vi "Dye Settings.vi"(6 "New Dye":bool, 8 "error in (no error)":errorcluster, 11 "Settings in":refnum<class "Settings.lvclass">=refnum) -> (0 "error out":errorcluster, 1 "Changed":bool, 2 "Pulse Sequence":T1(array[cluster])=[{"LED Name"="Cyan (488 nm)", "Pulse Length (s)"=0.1, "Delay Before (s)"=0.0, "Delay After (s)"=0.1, "Trigger Camera"=FALSE}, {"LED Name"="Red 2 (636 nm)", "Pulse Length (s)"=0.2, "Delay Before (s)"=0.0, "Delay After (s)"=0.1, "Trigger Camera"=TRUE}], 3 "Settings out":refnum<class "Settings.lvclass">)   [LabVIEW 2010, in "Settings.lvclass"]
uses:
  Settings.lvclass
  Settings.lvclass/Settings.ctl
panel:
  in  "# Pulses":i32=5 min=1 max=100
  out "Input OK":bool
  in  "Dye Name":string="Alexa 488"
  in  "Exposure (s)":dbl=0.2 min=0.0001 max=5.0
  in  "Delay After (s) 2":dbl=0.1 min=0.001 max=10.0 step=0.001
  in  "Pulse Length (s) 2":dbl=0.2 min=0.001 max=10.0 step=0.001
  in  "Delay Before (s) 2":dbl min=0.0 max=10.0 step=0.001
  in  "Delay After (s)":dbl=0.1 min=0.001 max=10.0 step=0.001
  in  "Pulse Length (s)":dbl=0.1 min=0.001 max=10.0 step=0.001
  in  "Delay Before (s)":dbl min=0.0 max=10.0 step=0.001
  out "XY Graph":cluster{dbl[], dbl[]}[](graph)=[{[0.0, 0.0, 0.0, 0.1, 0.1, 1.7000000000000002], [0.0, 0.0, 1.0, 1.0, 0.0, 0.0]}, {[0.0, 0.2, 0.2, 0.4, 0.4, 0.5, 0.5, 0.5, 0.7, 0.7, 0.7999999999999999, 0.7999999999999999, 0.7999999999999999, 1.0, 1.0, 1.1, 1.1, 1.1, 1.3, 1.3, 1.4000000000000001, 1.4000000000000001, 1.4000000000000001, 1.6, 1.6, 1.7000000000000002], [0.0, 0.0, 1.0, 1.0, 0.0, 0.0, 0.0, 1.0, 1.0, 0.0, 0.0, 0.0, 1.0, 1.0, 0.0, 0.0, 0.0, 1.0, 1.0, 0.0, 0.0, 0.0, 1.0, 1.0, 0.0, 0.0]}, {[0.0, 0.2, 0.2, 0.4, 0.4, 0.5, 0.5, 0.5, 0.7, 0.7, 0.7999999999999999, 0.7999999999999999, 0.7999999999999999, 1.0, 1.0, 1.1, 1.1, 1.1, 1.3, 1.3, 1.4000000000000001, 1.4000000000000001, 1.4000000000000001, 1.6, 1.6, 1.7000000000000002], [0.0, 0.0, 1.0, 1.0, 0.0, 0.0, 0.0, 1.0, 1.0, 0.0, 0.0, 0.0, 1.0, 1.0, 0.0, 0.0, 0.0, 1.0, 1.0, 0.0, 0.0, 0.0, 1.0, 1.0, 0.0, 0.0]}]
  in  "Cancel":bool
  in  "OK Button":bool
  in  "Emission Filter:":string(combo)="0"
  in  "Second Pulse:":string(combo)="Red 2 (636 nm)"
  in  "First Pulse:":string(combo)="Cyan (488 nm)"
  # "Dye Settings"
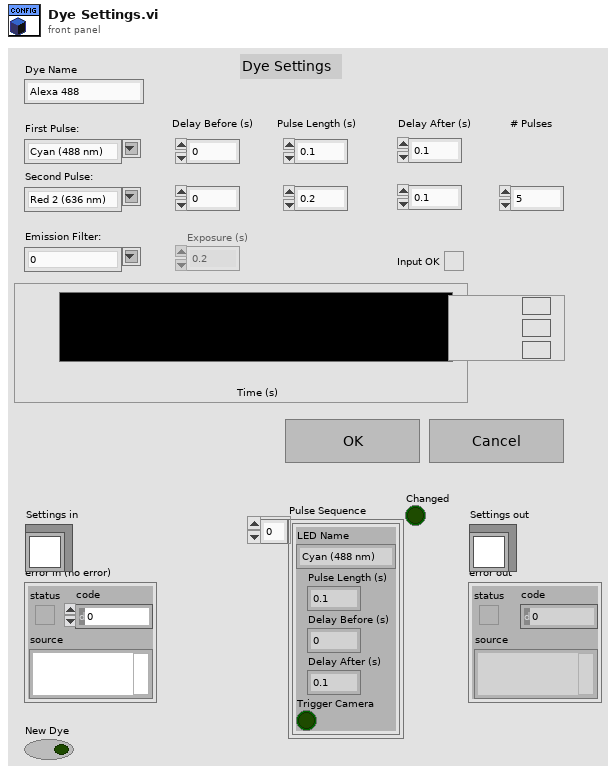
[diagram p1: front panel]
types:
  T1 = cluster{"LED Name":string, "Pulse Length (s)":dbl, "Delay Before (s)":dbl, "Delay After (s)":dbl, "Trigger Camera":bool}[]
  T2 = cluster{"Dye Name":string, "Pulse Sequence":cluster{"LED Name":string, "Pulse Length (s)":dbl, "Delay Before (s)":dbl, "Delay After (s)":dbl, "Trigger Camera":bool}[], "Emission Filter":i16, "Exposure (s)":dbl, "Yellow Select":bool, "# Pulses":i32}[]
  T3 = cluster{"Color":string, "DLL LED Num":i32, "Wavelength":i32, "Counter Name":string, "GRN_YEL":i32, "Yellow Select":i32, "Yellow Select Line":string}[]
  T4 = cluster{"Color":string, "Wavelength":i32, "Wheel Position":i32}[]
  T5 = cluster{"Dye Name":string, "Pulse Sequence":cluster{"LED Name":string, "Pulse Length (s)":dbl, "Delay Before (s)":dbl, "Delay After (s)":dbl, "Trigger Camera":bool}[], "Emission Filter":i16, "Exposure (s)":dbl, "Yellow Select":bool, "# Pulses":i32}
  T6 = cluster{"LED Name":string, "Pulse Length (s)":dbl, "Delay Before (s)":dbl, "Delay After (s)":dbl, "Trigger Camera":bool}
  T7 = cluster{"Dye Name":string, "Pulse Sequence":cluster{"LED Name":string, "Pulse Length (s)":dbl, "Delay Before (s)":dbl, "Delay After (s)":dbl, "Trigger Camera":bool}[], i32, "Exosure new (s)":dbl, "Yellow Select":bool, "# Pulses":i32}
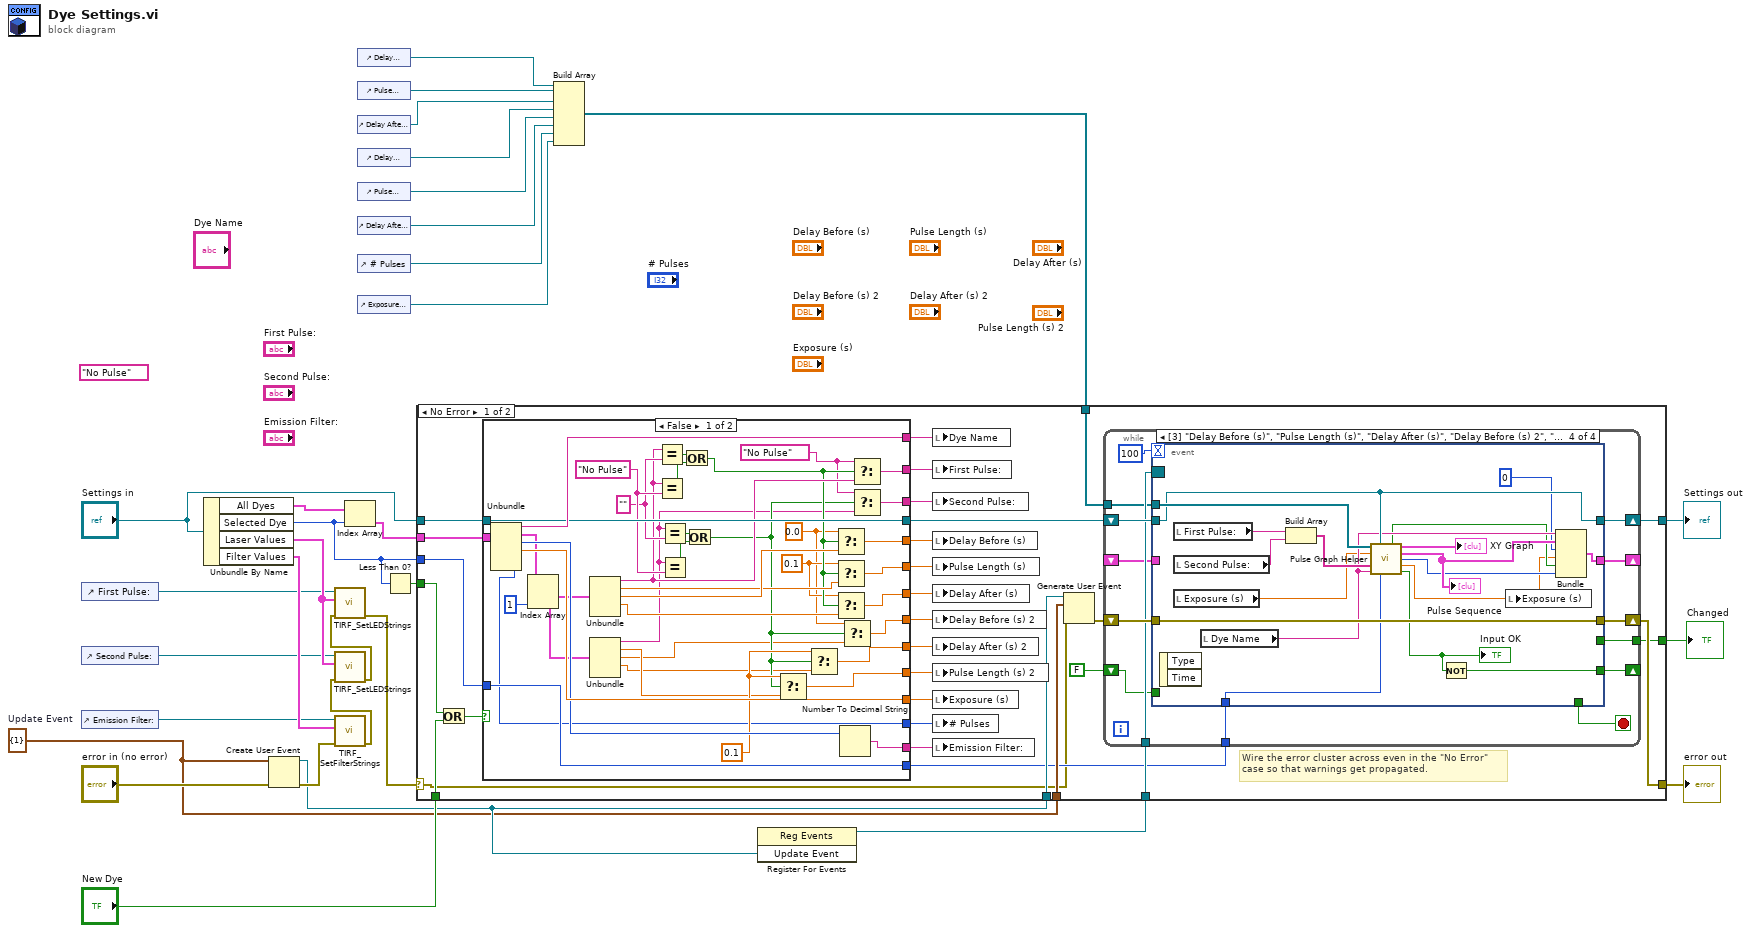
[diagram p0: block diagram]
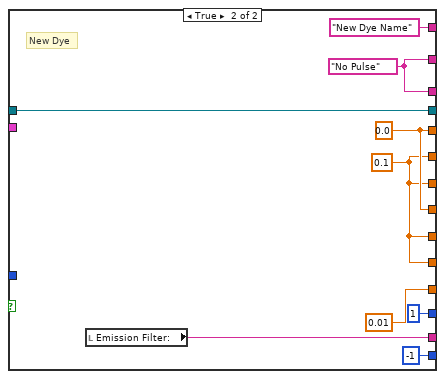
[diagram p2: hidden frame]
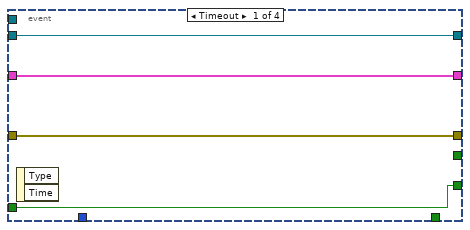
[diagram p3: hidden frame]
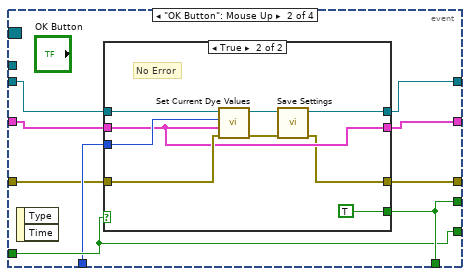
[diagram p4: hidden frame]
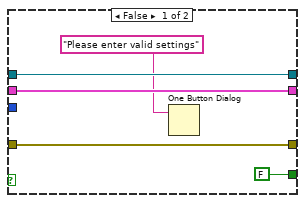
[diagram p5: hidden frame]
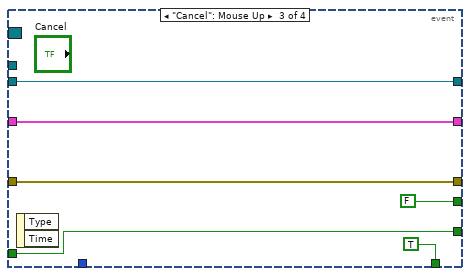
[diagram p6: hidden frame]
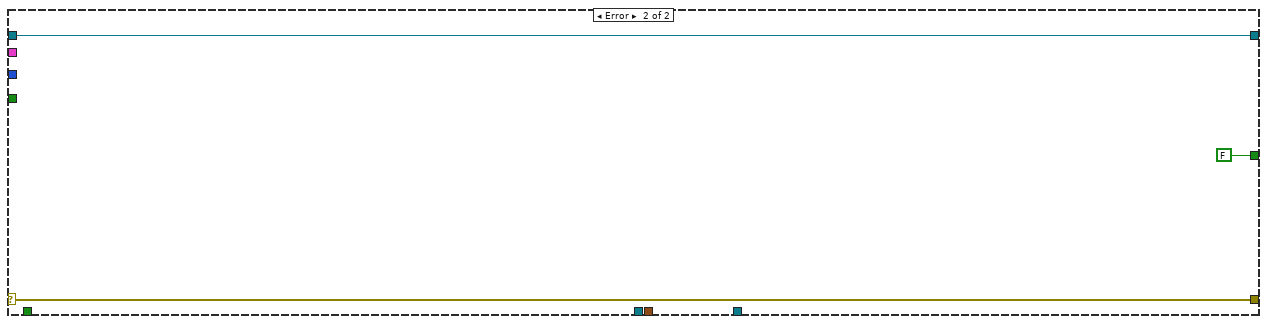
[diagram p7: hidden frame]
diagram:
  (unwired) "No Pulse" ("Second Pulse:")
  w15 = cluster{"index":i32} {"index"=1}  # Update Event
  n1 = control-ref of="First Pulse:"() -> (w27:refnum<vi>)
  n2 = control-ref of="Second Pulse:"() -> (w26:refnum<vi>)
  n3 = control-ref of="Emission Filter:"() -> (w25:refnum<vi>)
  n4 = Unbundle By Name("Settings in") -> ("All Dyes"=w8:T2, "Selected Dye"=w6:i32, "Laser Values"=w29:T3, "Filter Values"=w28:T4)
  n5 = Create User Event(user event datatype=w15, error in="error in (no error)") -> (user event=w16:refnum<user-event>, error out=w18:errorcluster)
  n6 = call "TIRF_SetFilterStrings.vi"("error in (no error)"=w18, "Filter Values"=w28, "Select Filter:"=w25) -> ("error out"=w24:errorcluster)  [unwired: 8 in]
  n7 = call "TIRF_SetLEDStrings.vi"("error in (no error)"=w24, "LED Values"=w29, "Select Filter:"=w26) -> ("error out"=w23:errorcluster)  [unwired: 8 in]
  n8 = call "TIRF_SetLEDStrings.vi"("error in (no error)"=w23, "LED Values"=w29, "Select Filter:"=w27) -> ("error out"=w22:errorcluster)  [unwired: 8 in]
  n9 = Index Array(array=w8, index=w6) -> (element=w7:T5)
  n10 = control-ref of="Delay Before (s)"() -> (w14:refnum<vi>)
  n11 = control-ref of="Pulse Length (s)"() -> (w13:refnum<vi>)
  n12 = control-ref of="Delay After (s)"() -> (w12:refnum<vi>)
  n13 = control-ref of="Delay Before (s) 2"() -> (w11:refnum<vi>)
  n14 = control-ref of="Pulse Length (s) 2"() -> (w4:refnum<vi>)
  n15 = control-ref of="Delay After (s) 2"() -> (w3:refnum<vi>)
  n16 = control-ref of="# Pulses"() -> (w2:refnum<vi>)
  n17 = control-ref of="Exposure (s)"() -> (w1:refnum<vi>)
  n18 = Less Than 0?(x=w6) -> (x < 0?=w5:bool)
  n19 = Build Array(w14, w13, w12, w11, w4, w3, w2, w1) -> (w10:refnum<vi>[])
  n20 = register-events(w16) -> (reference out=w17:refnum<event-registration>)  [unwired: 2 in, 1 out]
  n21 = case shown="No Error" w22 {
    selector: w22 -> [w35 w178]
    tunnel: [w49 w178] -> w31
    tunnel: [w61 w177] -> w30
    tunnel: "Settings in" -> [w34 w177]
    tunnel: "New Dye" -> [w42 _]
    tunnel: w17 -> [w44 _]
    tunnel: w16 -> [w46 _]
    tunnel: w15 -> [w45 _]
    tunnel: w10 -> [w43 _]
    tunnel: [w38 FALSE] -> w9
    tunnel: w6 -> [w37 _]
    tunnel: w7 -> [w36 _]
    tunnel: w5 -> [w33 _]
    frame No Error {
      # "Wire the error cluster across even in the \"No Error\"\ncase so that warnings get propagated."
      n22 = Or(x=w33, y=w42) -> (x .or. y?=w41:bool)
      n23 = case shown="False" w41 {
        tunnel: w34 -> [w93 w105]
        tunnel: [w93 w105] -> w60
        tunnel: [w99 w110] -> w59
        tunnel: [w68 w104] -> w48
        tunnel: [w84 w104] -> w58
        tunnel: [w98 "New Dye Name" ("Dye Name")] -> w57
        tunnel: [w81 w108] -> w56
        tunnel: [w74 w108] -> w55
        tunnel: [w80 w107] -> w54
        tunnel: [w78 w107] -> w53
        tunnel: [w72 w107] -> w52
        tunnel: [w73 w107] -> w51
        tunnel: [w101 0.01 ("Delay Before (s)")] -> w50
        tunnel: w36 -> [w92 _]
        tunnel: [w91 -1 ("Selected Dye")] -> w40
        tunnel: w37 -> [w91 _]
        tunnel: [w62 1 ("# Pulses")] -> w32
        frame False {
          w71 = 0.1 ("Delay Before (s)")
          w75 = 0.1 ("Delay Before (s)")
          w70 = 0.0 ("Delay Before (s)")
          w69 = "No Pulse" ("Second Pulse:")
          w86 = "No Pulse" ("y")
          w85 = "" ("y")
          n24 = Unbundle(w92) -> ("Dye Name"=w98:string, "Pulse Sequence"=w97:T1, "Emission Filter"=w100:i16, "Exposure (s)"=w101:dbl, "# Pulses"=w62:i32)  [unwired: 1 out]
          n25 = Index Array(array=w97, index #2=1 ("index")) -> (element #1=w96:T6, element #2=w94:T6)  [unwired: 1 in]
          n26 = Unbundle(w96) -> ("LED Name"=w83:string, "Pulse Length (s)"=w77:dbl, "Delay Before (s)"=w82:dbl, "Delay After (s)"=w79:dbl)  [unwired: 1 out]
          n27 = Unbundle(w94) -> ("LED Name"=w66:string, "Pulse Length (s)"=w65:dbl, "Delay Before (s)"=w64:dbl, "Delay After (s)"=w63:dbl)  [unwired: 1 out]
          n28 = Equal?(x=w83, y=w85) -> (x = y?=w90:bool)
          n29 = Equal?(x=w83, y=w86) -> (x = y?=w89:bool)
          n30 = Equal?(x=w66, y=w85) -> (x = y?=w88:bool)
          n31 = Equal?(x=w66, y=w86) -> (x = y?=w87:bool)
          n32 = Or(x=w90, y=w89) -> (x .or. y?=w76:bool)
          n33 = Or(x=w88, y=w87) -> (x .or. y?=w67:bool)
          n34 = Select(t=w71, s=w67, f=w65) -> (s? t:f=w73:dbl)
          n35 = Select(t=w71, s=w67, f=w63) -> (s? t:f=w72:dbl)
          n36 = Select(t=w70, s=w76, f=w82) -> (s? t:f=w81:dbl)
          n37 = Select(t=w75, s=w76, f=w77) -> (s? t:f=w80:dbl)
          n38 = Select(t=w75, s=w76, f=w79) -> (s? t:f=w78:dbl)
          n39 = Number To Decimal String(number=w100) -> (decimal integer string=w99:string)  [unwired: 1 in]
          n40 = Select(t=w70, s=w67, f=w64) -> (s? t:f=w74:dbl)
          n41 = Select(t=w69, s=w76, f=w83) -> (s? t:f=w84:string)
          n42 = Select(t=w69, s=w67, f=w66) -> (s? t:f=w68:string)
        }
        frame True {
          w104 = "No Pulse" ("Second Pulse:")
          w107 = 0.1 ("Delay Before (s)")
          w108 = 0.0 ("Delay Before (s)")
          # "New Dye"
          n43 = local read "Emission Filter:"() -> (w110:string)
        }
      }
      n44 = local write "Dye Name"(w57) -> ()
      n45 = local write "First Pulse:"(w58) -> ()
      n46 = local write "Second Pulse:"(w48) -> ()
      n47 = local write "Delay Before (s)"(w56) -> ()
      n48 = local write "Pulse Length (s)"(w54) -> ()
      n49 = local write "Delay After (s)"(w53) -> ()
      n50 = local write "Delay Before (s) 2"(w55) -> ()
      n51 = local write "Delay After (s) 2"(w52) -> ()
      n52 = local write "Pulse Length (s) 2"(w51) -> ()
      n53 = local write "Exposure (s)"(w50) -> ()
      n54 = local write "# Pulses"(w32) -> ()
      n55 = local write "Emission Filter:"(w59) -> ()
      n56 = Generate User Event(user event=w46, event data cluster=w45, error in=w35) -> (error out=w47:errorcluster)  [unwired: 1 out]
      n57 = while {
        shift-right: [w122] -> w61
        shift-left: w60 -> [w123]
        shift-right: [w119] -> w49
        shift-left: w47 -> [w120]
        tunnel: w44 -> [w118]
        tunnel: w43 -> [w117]
        tunnel: w40 -> [w116]
        shift-right: [w115] -> _
        shift-left: FALSE ("Error?") -> [w114]
        tunnel: [w113] -> w38
        shift-right: [w112] -> _
        shift-left: _ -> [w111]
        stop <- w121 stop-if-true
        n58 = event shown="[3] \"Delay Before (s)\", \"Pulse Length (s)\", \"Delay After (s)\", \"Delay Before (s) 2\", \"Pulse Length (s) 2\", \"Delay After (s) 2\", \"Exposure (s)\", \"First Pulse:\", \"Second Pulse:\", \"Dye Name\", \"Emission Filter:\", \"# Pulses\": Value Change;  <Update Event>: User Event" {
          selector: w118 -> [_ _ _ _]
          dyn-events: _ -> [_ _ _ _]
          timeout: 100 -> [_ _ _ _]
          tunnel: w123 -> [w128 w135 w156 w168]
          tunnel: [w128 w134 w156 w168] -> w122
          tunnel: [_ w137 TRUE _] -> w121
          tunnel: w120 -> [w127 w131 w155 w174]
          tunnel: [w127 w130 w155 w174] -> w119
          tunnel: w117 -> [_ _ _ w170]
          tunnel: w116 -> [_ w133 _ w169]
          tunnel: [w126 w136 w153 w166] -> w115
          tunnel: w114 -> [w126 w136 w153 _]
          tunnel: [_ w137 FALSE _] -> w113
          tunnel: [w125 w129 w152 w163] -> w112
          tunnel: w111 -> [w125 w132 w152 _]
          event Timeout {
            n59 = event-data() -> ()  [unwired: 1 in, 2 out]
          }
          event "OK Button": Mouse Up {
            n60 = event-data() -> ()  [unwired: 1 in, 2 out]
            n61 = case shown="True" w136 {
              tunnel: [FALSE TRUE] -> w137
              tunnel: w135 -> [w141 w150]
              tunnel: [w141 w145] -> w134
              tunnel: w133 -> [_ w149]
              tunnel: w132 -> [w139 w147]
              tunnel: w131 -> [w140 w148]
              tunnel: [w140 w143] -> w130
              tunnel: [w139 w147] -> w129
              frame False {
                n62 = One Button Dialog(message="Please enter valid settings") -> ()  [unwired: 1 in, 1 out]
              }
              frame True {
                # "No Error"
                n63 = call-dynamic "Set Current Dye Values.vi"("error in (no error)"=w148, "Dye Settings"=w147, "index"=w149, "Settings in"=w150) -> ("error out"=w144:errorcluster, "Settings out"=w146:refnum<class "Settings.lvclass">)  [unwired: 6 in]
                n64 = call-dynamic "Save Settings.vi"("error in (no error)"=w144, "Settings in"=w146) -> ("error out"=w143:errorcluster, "Settings out"=w145:refnum<class "Settings.lvclass">)  [unwired: 8 in]
              }
            }
          }
          event "Cancel": Mouse Up {
            n65 = event-data() -> ()  [unwired: 1 in, 2 out]
          }
          event "Delay Before (s)", "Pulse Length (s)", "Delay After (s)", "Delay Before (s) 2", "Pulse Length (s) 2", "Delay After (s) 2", "Exposure (s)", "First Pulse:", "Second Pulse:", "Dye Name", "Emission Filter:", "# Pulses": Value Change; User Event {
            n66 = event-data() -> ()  [unwired: 1 in, 2 out]
            n67 = local read "First Pulse:"() -> (w173:string)
            n68 = local read "Second Pulse:"() -> (w172:string)
            n69 = local read "Exposure (s)"() -> (w162:dbl)
            n70 = local read "Dye Name"() -> (w165:string)
            n71 = Build Array(w173, w172) -> (w171:string[])
            n72 = call "Pulse Graph Helper.vi"("Puls Times"=w170, "Settings in"=w168, "Exosure (s)"=w162, "Pulse Names"=w171, "New Dye Name"=w165, "Selected Dye"=w169) -> ("Yellow Select"=w161:bool, "Graph"=→"XY Graph":cluster{dbl[], dbl[]}[], "Pulse Sequence"=w164:T1, "# Pulses"=w160:i32, "Exosure new (s)"=w158:dbl, "Error?"=w167:bool)  [unwired: 4 in]
            "Pulse Sequence" <- w164
            "Input OK" <- w167
            n73 = Not(x=w167) -> (.not. x?=w166:bool)
            n74 = local write "Exposure (s)"(w158) -> ()
            n75 = Bundle("Dye Name"=w165, "Pulse Sequence"=w164, 0, "Exosure new (s)"=w158, "Yellow Select"=w161, "# Pulses"=w160) -> (w163:T7)  [unwired: 1 in]
          }
        }
      }
    }
    frame Error {
    }
  }
  "error out" <- w31
  "Settings out" <- w30
  "Changed" <- w9
